vi "Example_DIO_TDC.vi"() -> ()   [LabVIEW 2013]
uses:
  Instance           4 23Saved   Example_DIO_TDC .vi
  Instance           5 23Saved   Example_DIO_TDC .vi
  Instance           7 23Saved   Example_DIO_TDC .vi
panel:
  in  "Histogram number":i8 min=0 max=3
  in  "Second line":i8=1 min=0 max=31
  in  "serialNumber TDC":string="0NODCNYX"
  in  "partNumber TDC":string="SD-PXE-TDC-H0002-1G"
  in  "serialNumber DIO":string="0NODCNPD"
  in  "partNumber DIO":string="SD-PXE-DIO-H0002-128"
  out "errorOut TDC":errorcluster
  in  "First line":i8 min=0 max=31
  in  "nPort":i32(ring) items=["Port 0", "Port 1"]
  out "Delay \n(Seconds)":dbl
  out "i":i32
  out "errorOut DIO":errorcluster
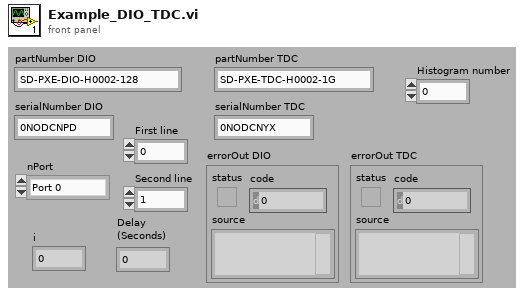
[diagram p1: front panel]
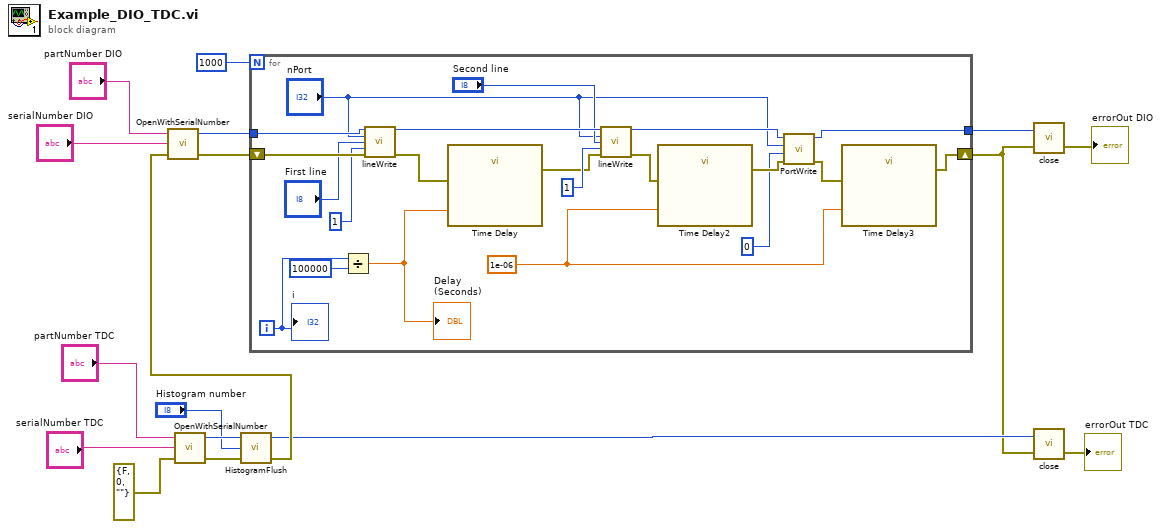
[diagram p0: block diagram]
diagram:
  n1 = call <vilib>:"OpenWithSerialNumber.vi"("errorIn"=errorcluster {"status"=FALSE, "code"=0, "source"=""}, "serialNumber"="serialNumber TDC", "partNumber"="partNumber TDC") -> ("errorOut"=w9:errorcluster, "moduleID"=w10:i32)  [unwired: 1 in]
  n2 = call <vilib>:"HistogramFlush.vi"("errorIn"=w9, "nHistogram"="Histogram number", "moduleID"=w10) -> ("errorOut"=w8:errorcluster, "moduleIDout"=w2:i32)  [unwired: 1 in]
  n3 = call <vilib>:"OpenWithSerialNumber.vi"("errorIn"=w8, "serialNumber"="serialNumber DIO", "partNumber"="partNumber DIO") -> ("errorOut"=w7:errorcluster, "moduleID"=w15:i32)  [unwired: 1 in]
  n4 = for {
    N: 1000 -> [_]
    tunnel: w15 -> [w36]
    tunnel: [w24] -> w4
    shift-right: [w27] -> w1
    shift-left: w7 -> [w35]
    i -> [w38]
    w18 = 1e-06 ("Delay Time (s)")
    n5 = Divide(x=w38, y=100000) -> (x/y=w19:dbl)
    "Delay \n(Seconds)" <- w19
    n6 = call <vilib>:"lineWrite.vi"("moduleID"=w36, "nPort"="nPort", "nLine"="First line", "lineValue"=1, "errorIn"=w35) -> ("moduleIDOut"=w31:i32, "errorOut"=w30:errorcluster)  [unwired: 9 in]
    n7 = call "Time Delay"("error in (no error)"=w30, "Delay Time (s)"=w19) -> ("error out"=w32:errorcluster)  [unwired: 9 in]
    n8 = call <vilib>:"lineWrite.vi"("moduleID"=w31, "nPort"="nPort", "nLine"="Second line", "lineValue"=i64 1 ("portValue"), "errorIn"=w32) -> ("moduleIDOut"=w25:i32, "errorOut"=w33:errorcluster)  [unwired: 9 in]
    n9 = call "Time Delay2"("error in (no error)"=w33, "Delay Time (s)"=w18) -> ("error out"=w23:errorcluster)  [unwired: 9 in]
    n10 = call <vilib>:"PortWrite.vi"("errorIn"=w23, "portValue"=i64 0, "nPort"="nPort", "moduleID"=w25) -> ("errorOut"=w22:errorcluster, "moduleIDOut"=w24:i32)  [unwired: 2 in]
    n11 = call "Time Delay3"("error in (no error)"=w22, "Delay Time (s)"=w18) -> ("error out"=w27:errorcluster)  [unwired: 9 in]
    "i" <- w38
  }
  n12 = call <vilib>:"close.vi"("errorIn"=w1, "moduleID"=w4) -> ("errorOut"=→"errorOut DIO":errorcluster)  [unwired: 1 in]
  n13 = call <vilib>:"close.vi"("errorIn"=w1, "moduleID"=w2) -> ("errorOut"=→"errorOut TDC":errorcluster)  [unwired: 1 in]
